vi "力特性 单点对称性.vi"(7 "单点压力":dbl, 8 "油压B":dbl[](array[numeric]), 9 "油压A":dbl[](array[numeric]), 10 "扭矩B":dbl[](array[numeric]), 11 "扭矩A":dbl[](array[numeric])) -> (3 "对称性":dbl)   [LabVIEW 2015, in "Logging.lvlib"]
uses:
  Logging.lvlib
  <vilib>/Analysis/1siggen.llb/Ramp Pattern by Samples.vi
  <vilib>/Analysis/NI_AALBase.lvlib
  <vilib>/gmath/NI_Gmath.lvlib
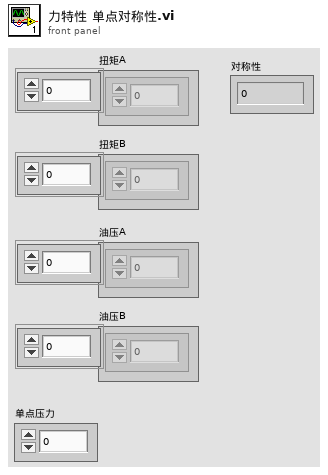
[diagram p1: front panel]
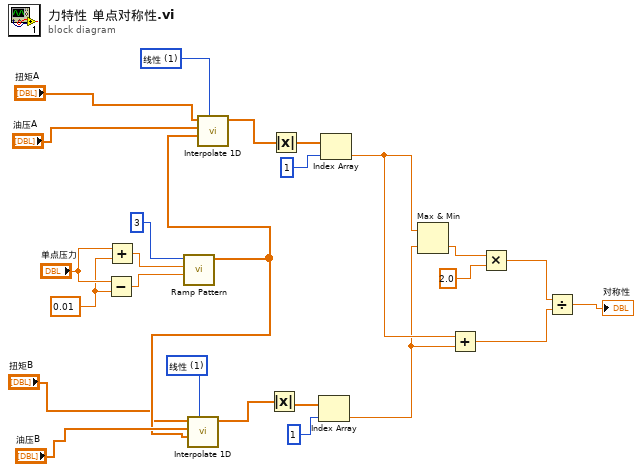
[diagram p0: block diagram]
diagram:
  w16 = 1 items=["最近", "线性", "样条", "cubic Hermite", "拉格朗日"] ("method")
  w19 = 1 items=["最近", "线性", "样条", "cubic Hermite", "拉格朗日"] ("method")
  w24 = 0.01 ("y")
  n1 = Subtract(x="单点压力", y=w24) -> (x-y=w22:dbl)
  n2 = Add(x="单点压力", y=w24) -> (x+y=w23:dbl)
  n3 = call-poly <vilib>:"Ramp Pattern.vi"("start"=w22, "end"=w23, "samples"=3) -> ("Ramp Pattern"=w17:dbl[])  [unwired: 7 in, 1 out]
  n4 = call <vilib>:"Interpolate 1D.vi"("method"=w16, "xi"=w17, "X"="油压B", "Y"="扭矩B") -> ("yi"=w14:dbl[])  [unwired: 5 in, 2 out]
  n5 = call <vilib>:"Interpolate 1D.vi"("method"=w19, "xi"=w17, "X"="油压A", "Y"="扭矩A") -> ("yi"=w15:dbl[])  [unwired: 5 in, 2 out]
  n6 = Absolute Value(x=w14) -> (abs(x)=w11:dbl[])
  n7 = Absolute Value(x=w15) -> (abs(x)=w13:dbl[])
  n8 = Index Array(array=w11, index=1 ("索引")) -> (element=w6:dbl)
  n9 = Index Array(array=w13, index=1 ("索引")) -> (element=w7:dbl)
  n10 = Max & Min(x=w7, y=w6) -> (min(x,y)=w9:dbl)  [unwired: 1 out]
  n11 = Add(x=w7, y=w6) -> (x+y=w4:dbl)
  n12 = Multiply(x=w9, y=2.0) -> (x*y=w5:dbl)
  n13 = Divide(x=w5, y=w4) -> (x/y=→"对称性":dbl)
